vi "ChName_2_chanFB.vi"(11 "Channel Name":u16(ring) items=["A1", "A2", "A3", "A4", "A5", "A6", "A7", "A8", "B1", "B2", "B3", "B4", "B5", "B6", "B7", "B8", "C1", "C2", "C3", "C4", "C5", "C6", "C7", "C8"]) -> (2 "Channel Out":enum16{"1", "2", "3", "4", "5", "6", "7", "8"}(ring), 3 "Flowboard Out":enum16{"A", "B", "C"}(ring))   [LabVIEW 2016]
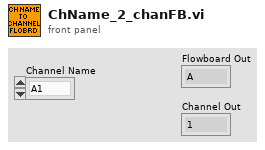
[diagram p1: front panel]
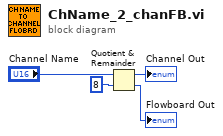
[diagram p0: block diagram]
diagram:
  n1 = Quotient & Remainder(x="Channel Name", y=u16 8) -> (x-y*floor(x/y)=→"Channel Out":u16, floor(x/y)=→"Flowboard Out":u16)
